vi "Close Transport.vi"(8 "error in (no error)":errorcluster, 11 "NotifierTransport":refnum<class "NotifierTransport.lvclass">) -> (0 "error out":errorcluster)   [LabVIEW 2017, in "NotifierTransport.lvclass"]
uses:
  NotifierTransport.lvclass
  NotifierTransport.lvclass/NotifierTransport.ctl
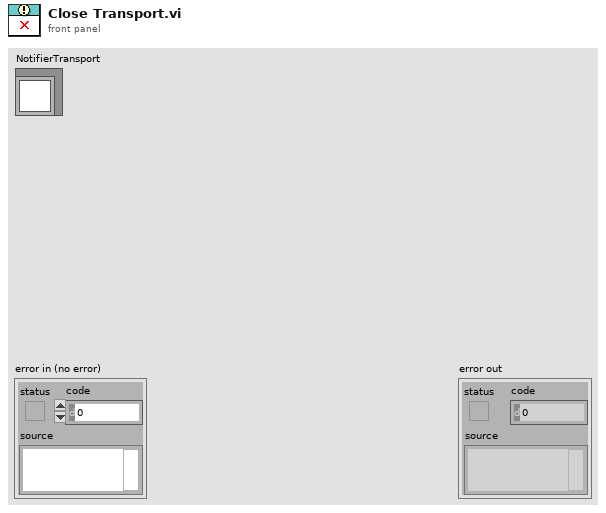
[diagram p1: front panel]
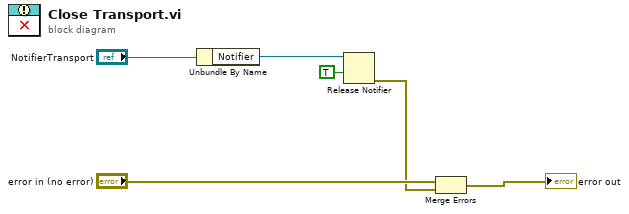
[diagram p0: block diagram]
diagram:
  n1 = Unbundle By Name("NotifierTransport") -> ("Notifier"=w3:refnum<notifier>)
  n2 = Release Notifier(notifier=w3, force destroy? (F)=TRUE) -> (error out=w1:errorcluster)  [unwired: 1 in, 2 out]
  n3 = Merge Errors("error in (no error)", w1) -> (→"error out":errorcluster)
